vi "Excel Format Image.vi"(0 "report in":refnum<class "NI_report.lvclass">, 1 "scale factor (1)":sgl=1.0 format="%.2f", 2 "measurement system":u16(ring) caption="measurement system (US)", 5 "picture index (-1)":i16=-1, 7 "height (-1)":sgl=-1.0 format="%.2f", 9 "width (-1)":sgl=-1.0 format="%.2f", 11 "error in (no error)":errorcluster, 12 "color type (auto)":i32(ring)=1 items=["msoPictureMixed"=-2, "msoPictureAutomatic"=1, "msoPictureGrayscale"=2, "msoPictureBlackAndWhite"=3, "msoPictureWatermark"=4]) -> (4 "report out":refnum<class "NI_report.lvclass">, 15 "error out":errorcluster)   [LabVIEW 2016, in "NI_Excel.lvclass"]
doc: "Formats the image specified by <B>picture index</B>. You can resize the image or modify its <B>color type</B>."
uses:
  <vilib>/Utility/NIReport.llb/Excel/NI_Excel.lvclass
  <vilib>/Utility/NIReport.llb/NI_report.lvclass
  C:/Program Files (x86)/National Instruments/LabVIEW 2016/vi.lib/Utility/NIReport.llb/NI_report.lvclass
  <vilib>/Utility/NIReport.llb/Excel/NI_Excel.lvclass/NI_Excel.ctl
  <vilib>/Utility/NIReport.llb/NI_ReportGenerationCore.lvlib
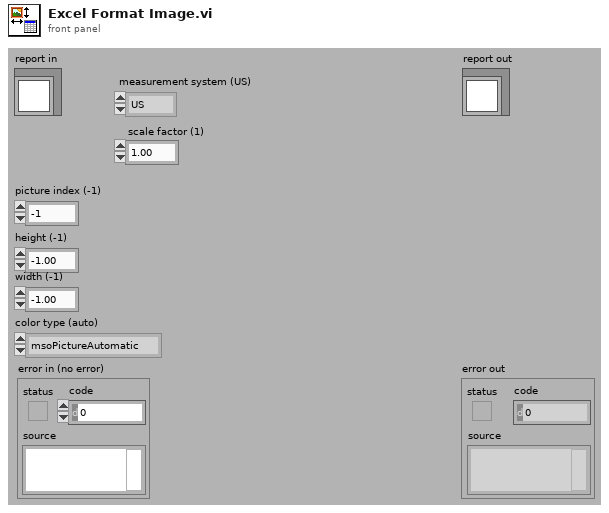
[diagram p1: front panel]
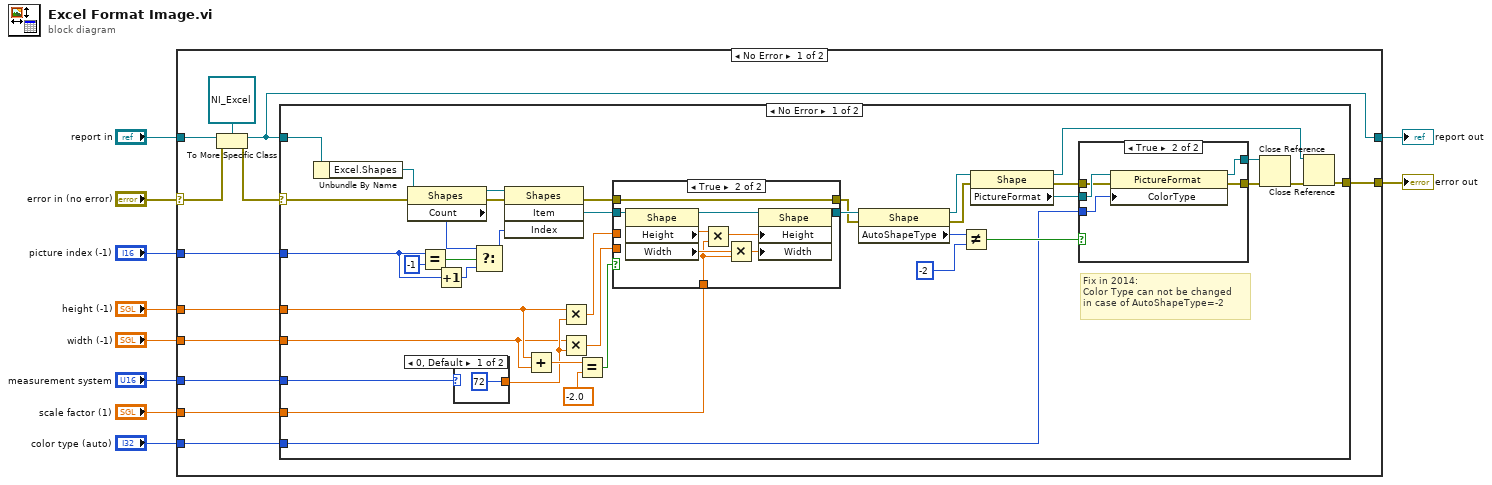
[diagram p0: block diagram]
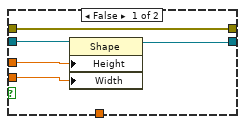
[diagram p3: hidden frame]
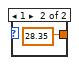
[diagram p4: hidden frame]
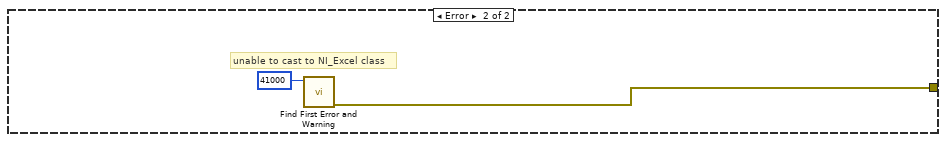
[diagram p5: hidden frame]
diagram:
  n1 = case shown="No Error" "error in (no error)" {
    selector: "error in (no error)" -> [w11 w87]
    tunnel: [w16 w87] -> w9
    tunnel: [w13 w86] -> w7
    tunnel: "report in" -> [w14 w86]
    tunnel: "picture index (-1)" -> [w22 _]
    tunnel: "height (-1)" -> [w21 _]
    tunnel: "width (-1)" -> [w20 _]
    tunnel: "measurement system" -> [w19 _]
    tunnel: "scale factor (1)" -> [w18 _]
    tunnel: "color type (auto)" -> [w17 _]
    frame No Error {
      n2 = To More Specific Class(target class=refnum<class "NI_Excel.lvclass"> refnum ("report in"), reference=w14, error in=w11) -> (specific class reference=w13:refnum<class "NI_Excel.lvclass">, error out=w12:errorcluster)
      n3 = case shown="No Error" w12 {
        selector: w12 -> [w38 _]
        tunnel: w22 -> [w44 _]
        tunnel: w21 -> [w43 _]
        tunnel: w20 -> [w42 _]
        tunnel: w19 -> [w41 _]
        tunnel: w18 -> [w40 _]
        tunnel: w17 -> [w28 _]
        tunnel: [w23 w84] -> w16
        tunnel: w13 -> [w39 _]
        frame No Error {
          # "Fix in 2014:\nColor Type can not be changed\nin case of AutoShapeType=-2"
          n4 = Unbundle By Name(w39) -> ("Excel.Shapes"=w60:refnum<k7>)
          n5 = property class="Shapes"(reference=w60, error in=w38) -> (reference out=w52:refnum<k7>, error out=w46:errorcluster, "Count"=w50:i32)
          n6 = Equal?(x=w44, y=i16 -1) -> (x = y?=w47:bool)
          n7 = Increment(x=w44) -> (x+1=w49:i16)
          n8 = case shown="0, Default" w41 {
            tunnel: [72 28.35] -> w55
            frame 0, Default {
            }
            frame 1 {
            }
          }
          n9 = Select(t=w50, s=w47, f=w49) -> (s? t:f=w51:i32)
          n10 = invoke class="Shapes" method="Item"(reference=w52, error in=w46, "Index"=w51) -> (error out=w56:errorcluster, "Item"=w45:refnum<k7>)  [unwired: 1 in, 2 out]
          n11 = Add(x=w43, y=w42) -> (x+y=w58:sgl)
          n12 = Multiply(x=w43, y=w55) -> (x*y=w53:dbl)
          n13 = Multiply(x=w42, y=w55) -> (x*y=w54:dbl)
          n14 = Equal?(x=w58, y=sgl -2.0) -> (x = y?=w57:bool)
          n15 = case shown="True" w57 {
            tunnel: w45 -> [w72 w81]
            tunnel: [w68 w78] -> w37
            tunnel: w53 -> [w71 _]
            tunnel: w54 -> [w70 _]
            tunnel: w56 -> [w69 w80]
            tunnel: [w69 w80] -> w36
            tunnel: w40 -> [_ w73]
            frame False {
              n16 = property class="Shape"(reference=w72, "Height"=w71, "Width"=w70) -> (reference out=w68:refnum<k7>)  [unwired: 1 in, 1 out]
            }
            frame True {
              n17 = property class="Shape"(reference=w81) -> (reference out=w79:refnum<k7>, "Height"=w77:sgl, "Width"=w76:sgl)  [unwired: 1 in, 1 out]
              n18 = Multiply(x=w77, y=w73) -> (x*y=w74:sgl)
              n19 = Multiply(x=w76, y=w73) -> (x*y=w75:sgl)
              n20 = property class="Shape"(reference=w79, "Height"=w74, "Width"=w75) -> (reference out=w78:refnum<k7>)  [unwired: 1 in, 1 out]
            }
          }
          n21 = property class="Shape"(reference=w37, error in=w36) -> (reference out=w32:refnum<k7>, error out=w31:errorcluster, "AutoShapeType"=w35:i32)
          n22 = Not Equal?(x=w35, y=-2) -> (x != y?=w33:bool)
          n23 = property class="Shape"(reference=w32, error in=w31) -> (reference out=w24:refnum<k7>, error out=w29:errorcluster, "PictureFormat"=w30:refnum<k7>)
          n24 = case shown="True" w33 {
            tunnel: w30 -> [w61 w67]
            tunnel: w29 -> [w62 w66]
            tunnel: w28 -> [_ w65]
            tunnel: [w62 w64] -> w27
            tunnel: [w61 w63] -> w26
            frame False {
            }
            frame True {
              n25 = property class="PictureFormat"(reference=w67, error in=w66, "ColorType"=w65) -> (reference out=w63:refnum<k7>, error out=w64:errorcluster)
            }
          }
          n26 = Close Reference(reference=w26, error in (no error)=w27) -> (error out=w25:errorcluster)
          n27 = Close Reference(reference=w24, error in (no error)=w25) -> (error out=w23:errorcluster)
        }
        frame Error {
          # "unable to cast to NI_Excel class"
          n28 = call <vilib>:"Find First Error and Warning.vi"("error code"=41000) -> ("error out"=w84:errorcluster)  [unwired: 2 in, 4 out]
        }
      }
    }
    frame Error {
    }
  }
  "error out" <- w9
  "report out" <- w7
